vi "总磷全局.vi"() -> ()   [LabVIEW 2016]
panel:
  in  "启动记录":string
  in  "启动模式":u16
  in  "总磷串口参数":T1={"VISA resource name"="", "baud rate (设置)"=115200, "unit ID"=1}
  out "启动运行次数":i32
  out "流程运行中":bool
  out "启动命令（模式）":string="空闲"
  in  "关键参数区输入":T2
  in  "测量数据区输入":T3 {"单位" items=["ug/L", "mg/L", "ppm", "mg/m3", "cm", "ppb", "ug/m3", "%", "nmol/mol", "umol/mol", "MPN/L", "MPN/100ml", "ng/m3", "NTU", "无量纲", "ms/cm", "us/cm", "℃", "mV", "万个/L"]}
  in  "状态告警区输入":T4
  out "运行状态":string
  in  "步骤时间/秒":T5={"步骤1时间"=2, "步骤2时间"=4, "步骤3时间"=2, "步骤4时间"=5, "步骤5时间"=6, "步骤6时间"=3, "步骤7时间"=4, "步骤8时间"=7, "步骤9时间"=8, "步骤10时间"=6}
  out "当前步骤":T6(ring)
  out "步骤运行时间/秒":i32
  out "流程结束":bool
  # "流程"
  # "流程步骤"
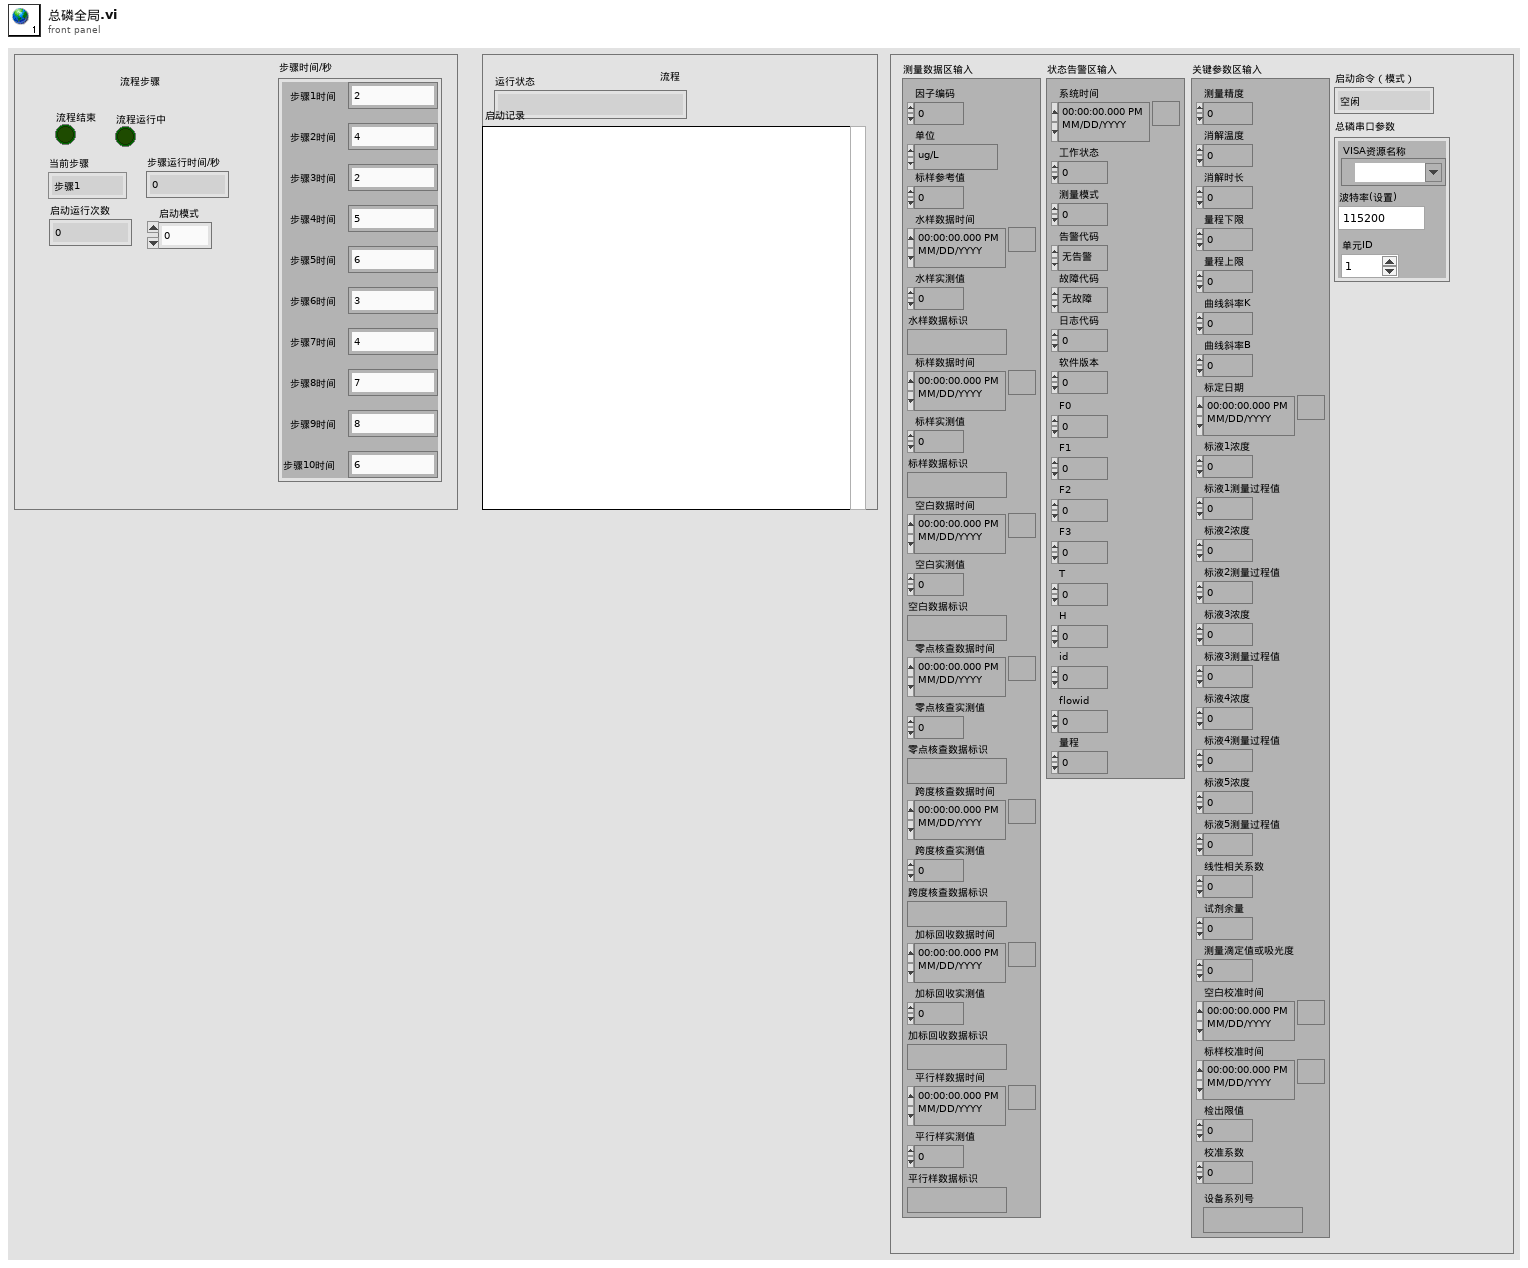
[diagram p1: front panel]
types:
  T1 = cluster{"VISA resource name":refnum<visa-resource-name>, "baud rate (设置)":u32, "unit ID":u8}
  T2 = cluster{"测量精度":u16, "消解温度":u16, "消解时长":u16, "量程下限":sgl, "量程上限":sgl, "曲线斜率K":sgl, "曲线斜率B":sgl, "标定日期":timestamp, "标液1浓度":sgl, "标液1测量过程值":sgl, "标液2浓度":sgl, "标液2测量过程值":sgl, "标液3浓度":sgl, "标液3测量过程值":sgl, "标液4浓度":sgl, "标液4测量过程值":sgl, "标液5浓度":sgl, "标液5测量过程值":sgl, "线性相关系数":sgl, "试剂余量":u32, "测量滴定值或吸光度":sgl, "空白校准时间":timestamp, "标样校准时间":timestamp, "检出限值":sgl, "校准系数":sgl, "设备系列号":string}
  T3 = cluster{"因子编码":u32, "单位":u16, "标样参考值":sgl, "水样数据时间":timestamp, "水样实测值":sgl, "水样数据标识":string, "标样数据时间":timestamp, "标样实测值":sgl, "标样数据标识":string, "空白数据时间":timestamp, "空白实测值":sgl, "空白数据标识":string, "零点核查数据时间":timestamp, "零点核查实测值":sgl, "零点核查数据标识":string, "跨度核查数据时间":timestamp, "跨度核查实测值":sgl, "跨度核查数据标识":string, "加标回收数据时间":timestamp, "加标回收实测值":sgl, "加标回收数据标识":string, "平行样数据时间":timestamp, "平行样实测值":sgl, "平行样数据标识":string}
  T4 = cluster{"系统时间":timestamp, "工作状态":u16, "测量模式":u16, "告警代码":enum16{"无告警", "缺试剂告警", "缺水样告警", "缺蒸馏水告警", "缺标液告警", "仪表漏液告警", "标定异常告警", "超量程告警", "加热异常", "低试剂预警", "超上限告警", "超下限告警", "仪表内部其他异常", "滴定异常告警", "电极异常告警", "量程切换告警", "参数设置告警", "PH电极电位异常", "电导率电极异常", "浊度光度异常", "溶解氧电极异常", "溶解氧光强异常", "温度异常告警", "PH异常告警", "溶解氧异常告警", "电导率异常告警", "浊度异常告警", "叶绿素异常告警", "藻密度异常告警", "蓝绿藻异常告警", "ORP异常告警", "氨氮异常告警", "清洁刷异常告警", "SD卡异常告警", "蓝牙异常告警", "Wifi异常告警", "流程异常告警"}, "故障代码":enum16{"无故障", "电机故障", "温度故障", "通讯故障", "滴定故障"}, "日志代码":u16, "软件版本":u16, "F0":sgl, "F1":sgl, "F2":sgl, "F3":sgl, "T":sgl, "H":sgl, "id":u16, "flowid":u16, "量程":u16}
  T5 = cluster{"步骤1时间":i32, "步骤2时间":i32, "步骤3时间":i32, "步骤4时间":i32, "步骤5时间":i32, "步骤6时间":i32, "步骤7时间":i32, "步骤8时间":i32, "步骤9时间":i32, "步骤10时间":i32}
  T6 = enum16{"步骤1", "步骤2", "步骤3", "步骤4", "步骤5", "步骤6", "步骤7", "步骤8", "步骤9", "步骤10"}
diagram:
